vi "GetParam.vi"(8 "error in (no error)":errorcluster caption="entrée d'erreur (pas d'erreur)", 11 "Cohen_Kappa_Score.lvclass":refnum<class "Cohen_Kappa_Score.lvclass">) -> (0 "error out":errorcluster caption="sortie d'erreur", 2 "cohen_kappa_score":T1={"labels"=[], "weights"="None", "sample_weight"=[]}, 3 "Cohen_Kappa_Score.lvclass":refnum<class "Cohen_Kappa_Score.lvclass">)   [LabVIEW 2020, in "Cohen_Kappa_Score.lvclass"]
doc: "Get Parameters"
uses:
  Cohen_Kappa_Score.lvclass
  Cohen_Kappa_Score.lvclass/Cohen_Kappa_Score.ctl
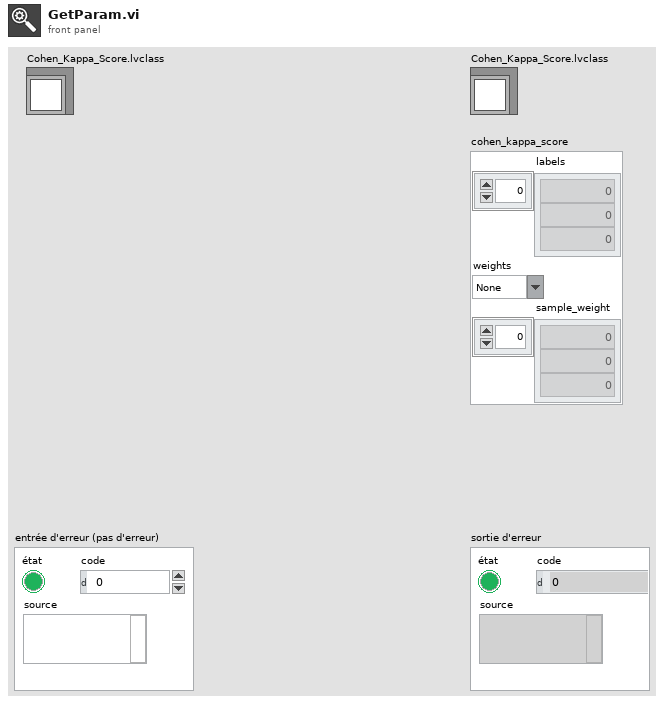
[diagram p1: front panel]
types:
  T1 = cluster{"labels":i32[], "weights":string, "sample_weight":dbl[]}
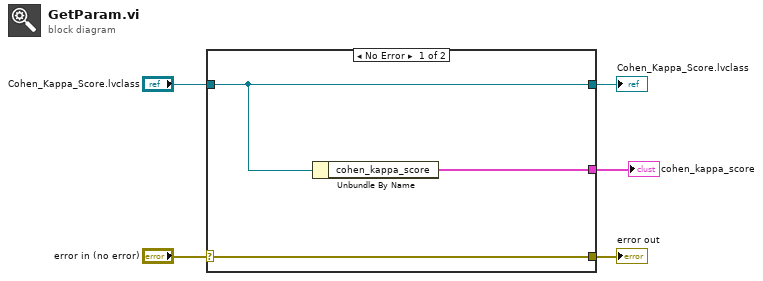
[diagram p0: block diagram]
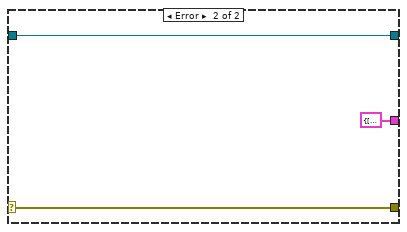
[diagram p2: hidden frame]
diagram:
  n1 = case shown="No Error" "error in (no error)" {
    selector: "error in (no error)" -> [w8 w10]
    tunnel: [w8 w10] -> w4
    tunnel: [w7 w11] -> w2
    tunnel: "Cohen_Kappa_Score.lvclass" -> [w7 w11]
    tunnel: [w6 T1 {"labels"=[], "weights"="", "sample_weight"=[]} ("cohen_kappa_score")] -> w1
    frame No Error {
      n2 = Unbundle By Name(w7) -> ("cohen_kappa_score"=w6:T1)
    }
    frame Error {
    }
  }
  "error out" <- w4
  "Cohen_Kappa_Score.lvclass" <- w2
  "cohen_kappa_score" <- w1
